vi "Save NIC Settings.vi"(7 "Network Interface:":u16, 8 "Error In":errorcluster, 11 "Install LV Data":T1) -> (0 "Error Out":errorcluster, 3 "Install LV Data":T1)   [LabVIEW 2014, in "LMH-LINX.lvlib"]
uses:
  <vilib>/MakerHub/LINX/LMH-LINX.lvlib
  <vilib>/MakerHub/LINX/Private/Utilties/Target Management/Install LV Data.ctl
  C:/Program Files (x86)/National Instruments/LabVIEW 2014/vi.lib/MakerHub/LINX/Resources/Renci.SshNet.dll
  Resources/Renci.SshNet.dll
  <vilib>/MakerHub/LINX/Private/Utilties/Target Management/Target Info.ctl
  <vilib>/MakerHub/LINX/Private/Utilties/Target Management/NIC Info.ctl
  <vilib>/MakerHub/LINX/Private/Utilties/Target Management/NIC Mode.ctl
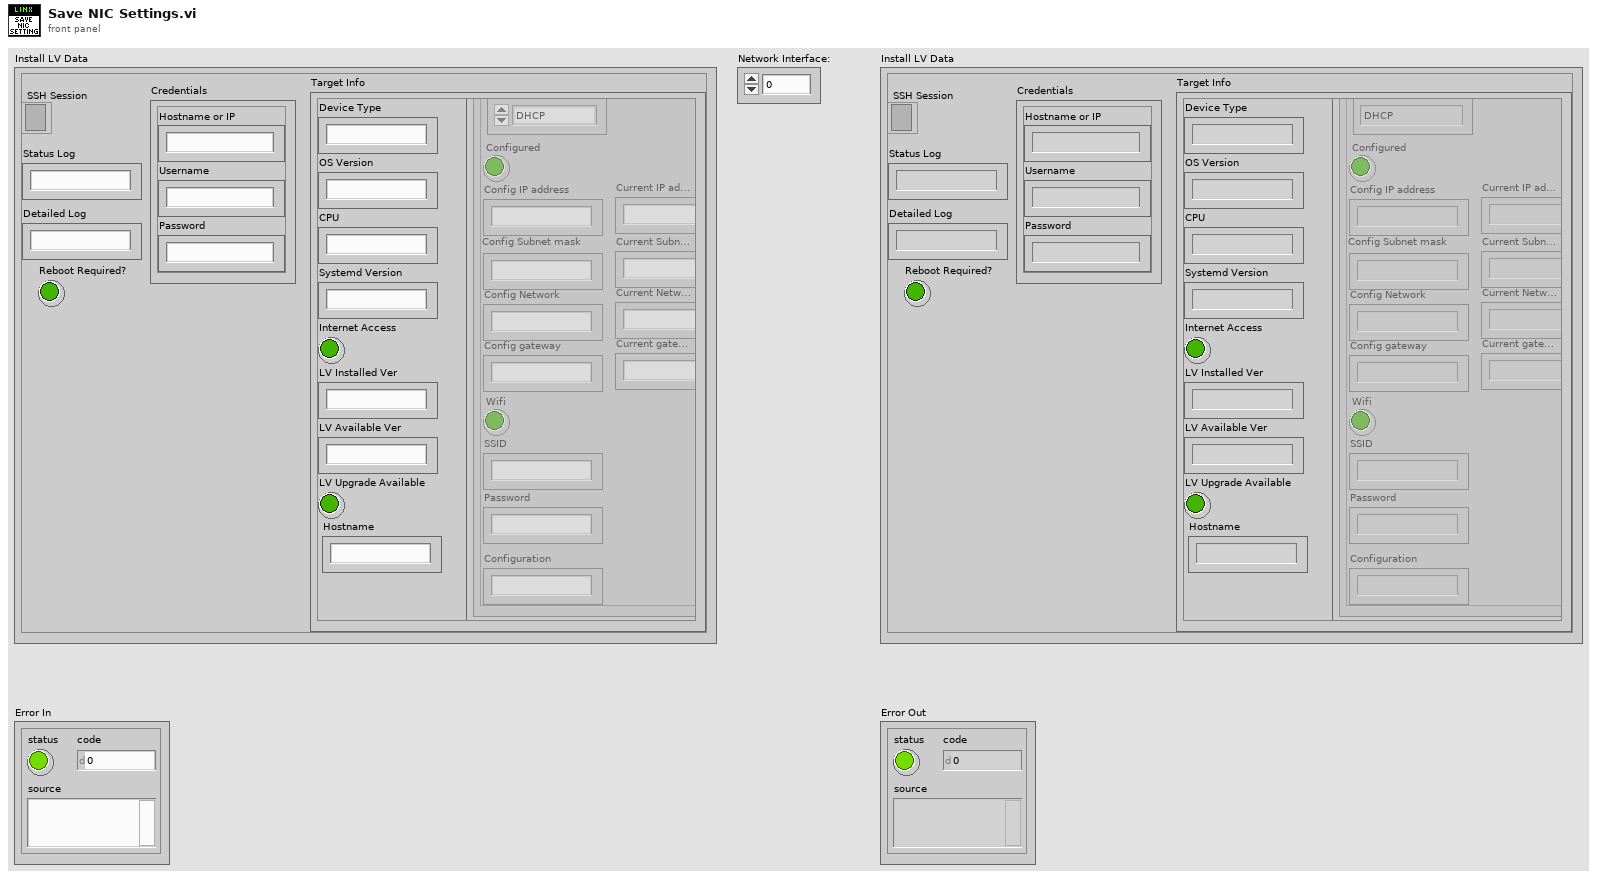
[diagram p1: front panel]
types:
  T1 = typedef "LMH-LINX.lvlib/Install LV Data.ctl" = cluster{"SSH Session":refnum<k24>, "Status Log":string, "Detailed Log":string, "Credentials":cluster{"Hostname or IP":string, "Username":string, "Password":string}, "Target Info":T2, "Reboot Required?":bool}
  T2 = typedef "LMH-LINX.lvlib/Target Info.ctl" = cluster{"OS Version":string, "CPU":string, "Systemd Version":string, "Internet Access":bool, "Device Type":string, "LV Installed Ver":string, "LV Available Ver":string, "LV Upgrade Available":bool, "Hostname":string, "NIC Info":T3[]}
  T3 = typedef "LMH-LINX.lvlib/NIC Info.ctl" = cluster{"Name":string, "NIC Mode":T4, "Configured":bool, "Config IP address":string, "Config Subnet mask":string, "Config Network":string, "Config gateway":string, "Wifi":bool, "SSID":string, "Password":string, "Configuration":string, "Current IP address":string, "Current Subnet mask":string, "Current gateway":string, "Current Network":string}
  T4 = typedef "LMH-LINX.lvlib/NIC Mode.ctl" = enum16{"DHCP", "Static", "Loopback"}
  T5 = typedef "LMH-LINX.lvlib/Network Settings Ctrl Refs.ctl" = cluster{"Hostname":refnum<vi>, "IP address":refnum<vi>, "Subnet mask":refnum<vi>, "Default Gateway":refnum<vi>, "SSID":refnum<vi>, "Password":refnum<vi>, "NIC Status":refnum<vi>, "Network Interface":refnum<vi>, "DCHP":refnum<vi>}
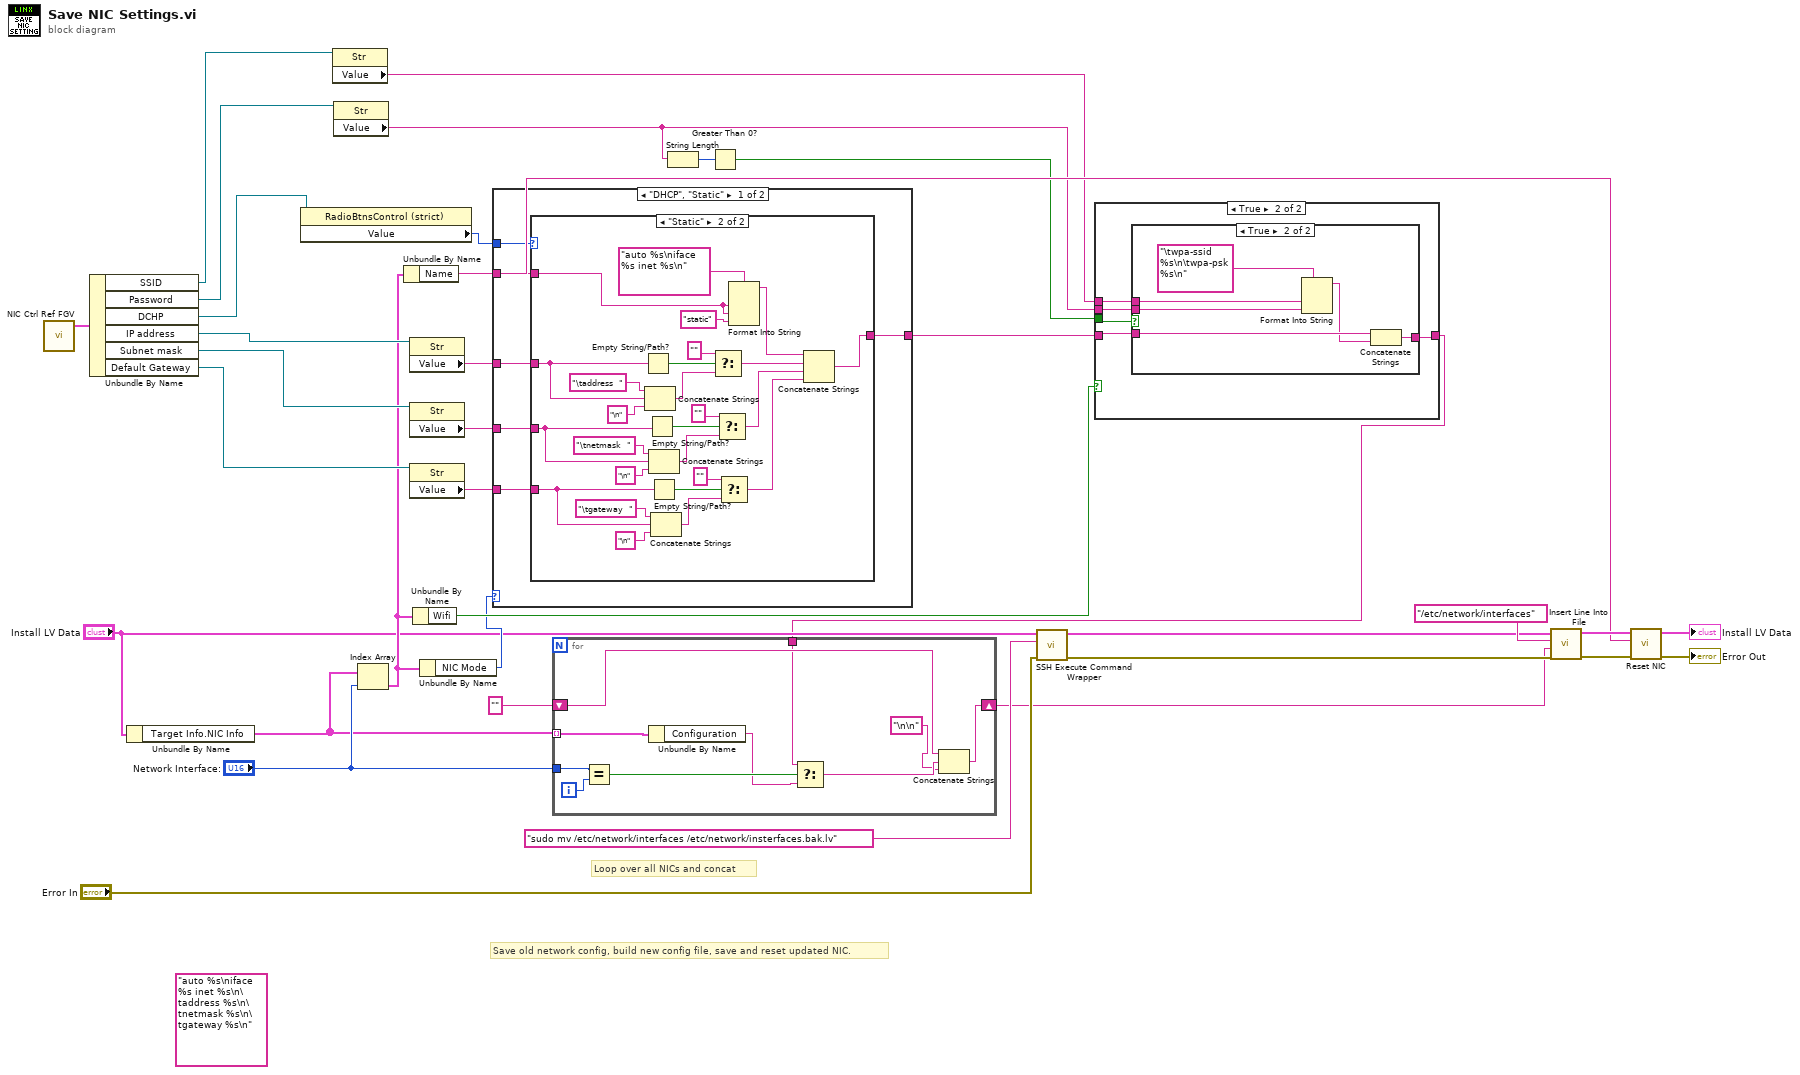
[diagram p0: block diagram]
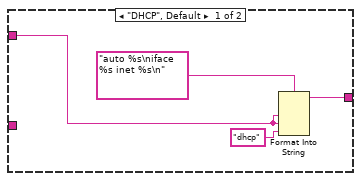
[diagram p2: hidden frame]
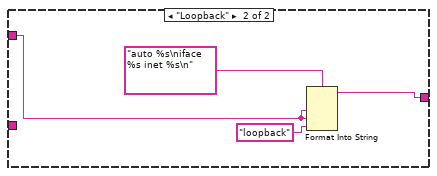
[diagram p3: hidden frame]
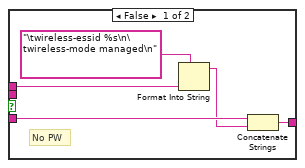
[diagram p5: hidden frame]
diagram:
  (unwired) "auto %s\niface %s inet %s\n\taddress %s\n\tnetmask %s\n\tgateway %s\n"
  # "Loop over all NICs and concat"
  # "Save old network config, build new config file, save and reset updated NIC."
  n1 = call <vilib>:"NIC Ctrl Ref FGV.vi"() -> ("Network Settings Ctrl Refs"=w27:T5)  [unwired: 4 in]
  n2 = Unbundle By Name(w27) -> ("SSID"=w20:refnum<vi>, "Password"=w19:refnum<vi>, "DCHP"=w28:refnum<vi>, "IP address"=w30:refnum<vi>, "Subnet mask"=w31:refnum<vi>, "Default Gateway"=w32:refnum<vi>)
  n3 = Unbundle By Name("Install LV Data") -> ("Target Info.NIC Info"=w10:T3[])
  n4 = property class="RadioBtnsControl (strict)"(reference=w28) -> ("Value"=w29:enum32{"DHCP", "Static"})  [unwired: 1 in, 2 out]
  n5 = property class="Str"(reference=w20) -> ("Value"=w18:string)  [unwired: 1 in, 2 out]
  n6 = property class="Str"(reference=w19) -> ("Value"=w17:string)  [unwired: 1 in, 2 out]
  n7 = Index Array(array=w10, index="Network Interface:") -> (element=w9:T3)
  n8 = Unbundle By Name(w9) -> ("Name"=w25:string)
  n9 = property class="Str"(reference=w30) -> ("Value"=w33:string)  [unwired: 1 in, 2 out]
  n10 = property class="Str"(reference=w31) -> ("Value"=w34:string)  [unwired: 1 in, 2 out]
  n11 = property class="Str"(reference=w32) -> ("Value"=w35:string)  [unwired: 1 in, 2 out]
  n12 = Unbundle By Name(w9) -> ("Wifi"=w12:bool)
  n13 = Unbundle By Name(w9) -> ("NIC Mode"=w8:T4)
  n14 = case shown="\"DHCP\", \"Static\"" w8 {
    tunnel: w35 -> [w41 _]
    tunnel: w34 -> [w40 _]
    tunnel: w33 -> [w39 _]
    tunnel: w29 -> [w38 _]
    tunnel: w25 -> [w37 w73]
    tunnel: [w36 w72] -> w21
    frame "DHCP", "Static" {
      n15 = case shown="\"Static\"" w38 {
        tunnel: [w43 w61] -> w36
        tunnel: w37 -> [w42 w69]
        tunnel: w39 -> [_ w64]
        tunnel: w40 -> [_ w52]
        tunnel: w41 -> [_ w51]
        frame "DHCP", Default {
          n16 = Format Into String(format string="auto %s\niface %s inet %s\n", w42, w42, "dhcp" ("input 2")) -> (resulting string=w43:string)  [unwired: 2 in, 1 out]
        }
        frame "Static" {
          n17 = Empty String/Path?(string/path=w64) -> (empty?=w66:bool)
          n18 = Concatenate Strings("\taddress  ", w64, "\n" ("string")) -> (w67:string)
          n19 = Empty String/Path?(string/path=w52) -> (empty?=w59:bool)
          n20 = Concatenate Strings("\tnetmask  ", w52, "\n" ("string")) -> (w58:string)
          n21 = Empty String/Path?(string/path=w51) -> (empty?=w54:bool)
          n22 = Concatenate Strings("\tgateway  ", w51, "\n" ("string")) -> (w55:string)
          n23 = Select(t="", s=w66, f=w67) -> (s? t:f=w62:string)
          n24 = Select(t="", s=w59, f=w58) -> (s? t:f=w50:string)
          n25 = Select(t="", s=w54, f=w55) -> (s? t:f=w49:string)
          n26 = Format Into String(format string="auto %s\niface %s inet %s\n", w69, w69, "static" ("input 2")) -> (resulting string=w63:string)  [unwired: 2 in, 1 out]
          n27 = Concatenate Strings(w63, w62, w50, w49) -> (w61:string)
        }
      }
    }
    frame "Loopback" {
      n28 = Format Into String(format string="auto %s\niface %s inet %s\n", w73, w73, "loopback" ("input 2")) -> (resulting string=w72:string)  [unwired: 2 in, 1 out]
    }
  }
  n29 = String Length(string=w17) -> (length=w16:i32)
  n30 = Greater Than 0?(x=w16) -> (x > 0?=w15:bool)
  n31 = call <vilib>:"SSH Execute Command Wrapper.vi"("Error In"="Error In", "Command"="sudo mv /etc/network/interfaces /etc/network/insterfaces.bak.lv", "Install LV Data in"="Install LV Data") -> ("Error Out"=w5:errorcluster, "Install LV Data out"=w2:T1)  [unwired: 6 in, 1 out]
  n32 = case shown="True" w12 {
    tunnel: [w76 w80] -> w3
    tunnel: w21 -> [w76 w79]
    tunnel: w18 -> [_ w81]
    tunnel: w17 -> [_ w77]
    tunnel: w15 -> [_ w78]
    frame False {
      # "Not Wifi...Move Along..."
    }
    frame True {
      n33 = case shown="True" w78 {
        tunnel: w81 -> [w85 w92]
        tunnel: [w84 w91] -> w80
        tunnel: w79 -> [w83 w90]
        tunnel: w77 -> [_ w88]
        frame False {
          # "No PW"
          n34 = Format Into String(format string="\twireless-essid %s\n\twireless-mode managed\n", w85) -> (resulting string=w82:string)  [unwired: 2 in, 1 out]
          n35 = Concatenate Strings(w83, w82) -> (w84:string)
        }
        frame True {
          n36 = Format Into String(format string="\twpa-ssid %s\n\twpa-psk %s\n", w92, w88) -> (resulting string=w89:string)  [unwired: 2 in, 1 out]
          n37 = Concatenate Strings(w90, w89) -> (w91:string)
        }
      }
    }
  }
  n38 = for {
    tunnel: "Network Interface:" -> [w102]
    tunnel: w10 -> [w97] mode=indexing
    shift-right: [w100] -> w1
    shift-left: "" ("string") -> [w99]
    tunnel: w3 -> [w96]
    i -> [w101]
    n39 = Equal?(x=w102, y=w101) -> (x = y?=w98:bool)
    n40 = Unbundle By Name(w97) -> ("Configuration"=w95:string)
    n41 = Select(t=w96, s=w98, f=w95) -> (s? t:f=w94:string)
    n42 = Concatenate Strings(w99, w94, "\n\n" ("string")) -> (w100:string)
  }
  n43 = call <vilib>:"Insert Line Into File.vi"("Error In"=w5, "Line"=w1, "File Path"="/etc/network/interfaces", "Install LV Data"=w2) -> ("Error Out"=w24:errorcluster, "Install LV Data"=w26:T1)  [unwired: 4 in, 2 out]
  n44 = call <vilib>:"Reset NIC.vi"("Error In"=w24, "NIC Name"=w25, "Install LV Data"=w26) -> ("Error Out"=→"Error Out":errorcluster, "Install LV Data out"=→"Install LV Data":T1)  [unwired: 7 in]
